vi "DRIVE_HOLD.vi"(10 "argv":string[](array[string]), 11 "args":u8) -> ()   [LabVIEW 2011]
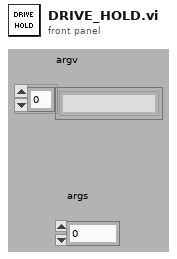
[diagram p1: front panel]
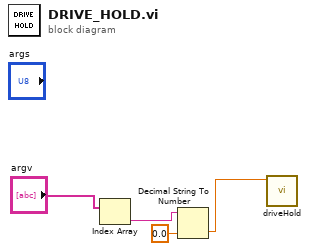
[diagram p0: block diagram]
diagram:
  n1 = Index Array(array="argv") -> (element=w3:string)  [unwired: 1 in]
  n2 = Decimal String To Number(string=w3, default (0L)=0.0 ("default (0 I32)")) -> (number=w2:dbl)  [unwired: 1 in, 1 out]
  n3 = call "driveHold.vi"("time"=w2) -> ()  [unwired: 11 in]
